vi "Main.vi"() -> ()   [LabVIEW 2018]
uses:
  Tank Class/Tank.lvclass
  Sensor Class/Sensor.lvclass
  Pump Class/Pump.lvclass
  Pump Class/Pump.lvclass/Pump.ctl
  Sensor Class/Sensor.lvclass/Sensor.ctl
  Tank Class/Tank.lvclass/Tank.ctl
  State Machines/Shared/Globals.vi
panel:
  out "Level 2":bool
  out "Level 1":bool
  out "Pump":bool
  in  "stop":bool
  out "Tank":dbl(slide) scale=0.0..100.0
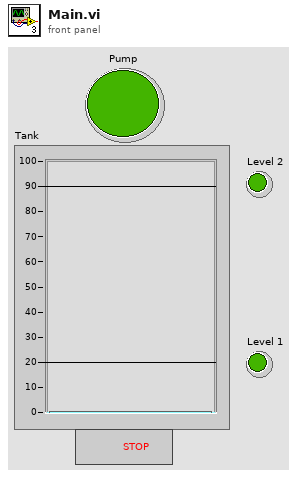
[diagram p1: front panel]
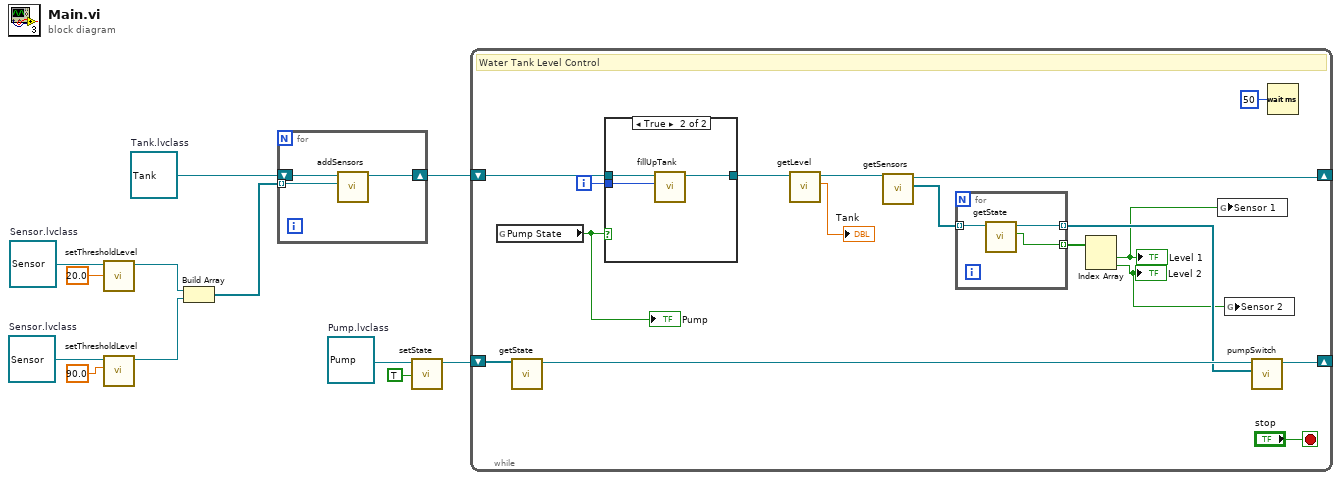
[diagram p0: block diagram]
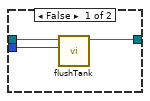
[diagram p2: hidden frame]
diagram:
  w3 = refnum<class "Pump.lvclass"> refnum  # Pump.lvclass
  w11 = refnum<class "Sensor.lvclass"> refnum  # Sensor.lvclass
  w10 = refnum<class "Sensor.lvclass"> refnum  # Sensor.lvclass
  w12 = refnum<class "Tank.lvclass"> refnum  # Tank.lvclass
  n1 = call "setThresholdLevel.vi"("Threshold Level"=20.0, "Sensor in"=w10) -> ("Sensor out"=w8:refnum<class "Sensor.lvclass">)  [unwired: 8 in, 1 out]
  n2 = call "setThresholdLevel.vi"("Threshold Level"=90.0, "Sensor in"=w11) -> ("Sensor out"=w7:refnum<class "Sensor.lvclass">)  [unwired: 8 in, 1 out]
  n3 = Build Array(w8, w7) -> (w4:refnum<class "Sensor.lvclass">[])
  n4 = for {
    shift-right: [w14] -> w9
    shift-left: w12 -> [w15]
    tunnel: w4 -> [w13] mode=indexing
    n5 = call "addSensors.vi"("Sensor.lvclass"=w13, "Tank in"=w15) -> ("Tank out"=w14:refnum<class "Tank.lvclass">)  [unwired: 8 in, 1 out]
  }
  n6 = call "setState.vi"("state"=TRUE, "Pump in"=w3) -> ("Pump out"=w2:refnum<class "Pump.lvclass">)  [unwired: 8 in, 1 out]
  n7 = while {
    shift-right: [w29] -> _
    shift-left: w2 -> [w30]
    shift-right: [w22] -> _
    shift-left: w9 -> [w27]
    i -> [w21]
    stop <- "stop" stop-if-true
    # "Water Tank Level Control"
    n8 = global read "Globals.vi" "Pump State"() -> (w18:bool)
    "Pump" <- w18
    n9 = call "getState.vi"("Pump in"=w30) -> ("Pump out"=w28:refnum<class "Pump.lvclass">)  [unwired: 8 in, 2 out]
    n10 = case shown="True" w18 {
      tunnel: [w34 w38] -> w32
      tunnel: w27 -> [w35 w37]
      tunnel: w21 -> [w33 w36]
      frame False {
        n11 = call "flushTank.vi"("Index"=w33, "Tank in"=w35) -> ("Tank out"=w34:refnum<class "Tank.lvclass">)  [unwired: 8 in, 1 out]
      }
      frame True {
        n12 = call "fillUpTank.vi"("Index"=w36, "Tank in"=w37) -> ("Tank out"=w38:refnum<class "Tank.lvclass">)  [unwired: 8 in, 1 out]
      }
    }
    n13 = call "getLevel.vi"("Tank in"=w32) -> ("Level"=→"Tank":dbl, "Tank out"=w20:refnum<class "Tank.lvclass">)  [unwired: 8 in, 1 out]
    n14 = call "getSensors.vi"("Tank in"=w20) -> ("Sensors"=w31:refnum<class "Sensor.lvclass">[], "Tank out"=w22:refnum<class "Tank.lvclass">)  [unwired: 8 in, 1 out]
    n15 = for {
      tunnel: w31 -> [w41] mode=indexing
      tunnel: [w40] -> w25 mode=indexing
      tunnel: [w39] -> w24 mode=indexing
      n16 = call "getState.vi"("Sensor in"=w41) -> ("State"=w39:bool, "Sensor out"=w40:refnum<class "Sensor.lvclass">)  [unwired: 8 in, 1 out]
    }
    n17 = Index Array(array=w24) -> (element #1=w17:bool, element #2=w16:bool)  [unwired: 2 in]
    "Level 1" <- w17
    "Level 2" <- w16
    n18 = global write "Globals.vi" "Sensor 1"(w17) -> ()
    n19 = global write "Globals.vi" "Sensor 2"(w16) -> ()
    n20 = call "pumpSwitch.vi"("Sensors"=w25, "Pump in"=w28) -> ("Pump out"=w29:refnum<class "Pump.lvclass">)  [unwired: 8 in, 1 out]
    n21 = Wait (ms)(milliseconds to wait=u32 50) -> ()  [unwired: 1 out]
  }
